vi "StartPythonEventLog.vi"(11 "Console Visibility":T1) -> (3 "Session ID out":T2 format="%x")   [LabVIEW 2018]
uses:
  <vilib>/Enthought/Python Integration Toolkit/api/Session ID.ctl
  <vilib>/Enthought/Python Integration Toolkit/api/Console Visibility.ctl
  Global Variables.vi
  <vilib>/Enthought/Python Integration Toolkit/Python Integration Toolkit.lvlib
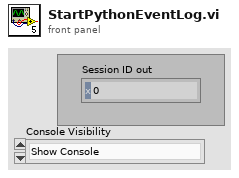
[diagram p1: front panel]
types:
  T1 = typedef "Python Integration Toolkit.lvlib/Console Visibility.ctl" = enum16{"Show Console", "Show Console While Running", "Hide Console"}
  T2 = typedef "Python Integration Toolkit.lvlib/Session ID.ctl" = u64
  T3 = enum16{"open", "replace", "create", "open or create", "replace or create", "replace or create with confirmation"}
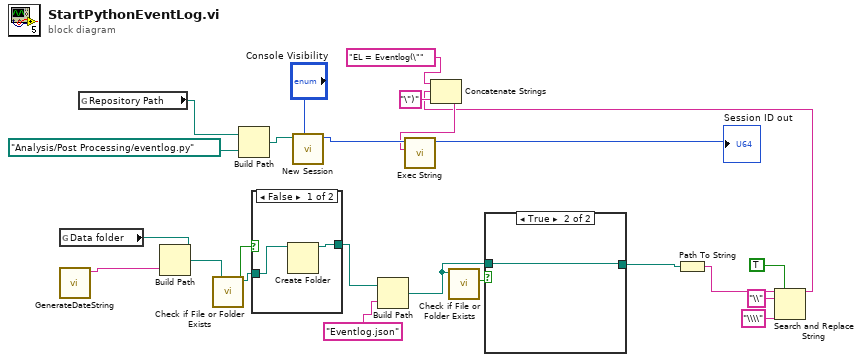
[diagram p0: block diagram]
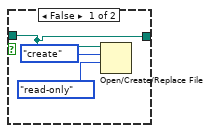
[diagram p2: hidden frame]
diagram:
  n1 = global read "Global Variables.vi" "Data folder"() -> (w18:path)
  n2 = call "GenerateDateString.vi"() -> ("String"=w19:string)  [unwired: 11 in]
  n3 = global read "Global Variables.vi" "Repository Path"() -> (w14:path)
  n4 = Build Path(base path=w18, name or relative path=w19) -> (appended path=w22:path)
  n5 = call <vilib>:"Check if File or Folder Exists.vi"("path"=w22) -> ("file or folder exists?"=w20:bool, "dup path"=w21:path)  [unwired: 8 in, 1 out]
  n6 = Build Path(base path=w14, name or relative path=path "Analysis/Post Processing/eventlog.py" ("vi path")) -> (appended path=w16:path)
  n7 = case shown="False" w20 {
    tunnel: w21 -> [w26 w27]
    tunnel: [w25 w27] -> w23
    frame False {
      n8 = Create Folder(path (use dialog)=w26) -> (created path=w25:path)  [unwired: 2 in, 2 out]
    }
    frame True {
    }
  }
  n9 = call <vilib>:"New Session.vi"("Console Visibility"="Console Visibility", "Path to Python Module (.py File)"=w16) -> ("Session ID out"=w10:T2)  [unwired: 8 in, 1 out]
  n10 = Build Path(base path=w23, name or relative path="Eventlog.json" ("string")) -> (appended path=w12:path)
  n11 = call <vilib>:"Check if File or Folder Exists.vi"("path"=w12) -> ("file or folder exists?"=w13:bool)  [unwired: 8 in, 2 out]
  n12 = case shown="True" w13 {
    tunnel: w12 -> [w30 w31]
    tunnel: [w30 w31] -> w11
    frame False {
      n13 = Open/Create/Replace File(file path (use dialog)=w30, operation (0:open)=T3."create", access (0:read/write)=enum16{"read/write", "read-only", "write-only"}."read-only") -> ()  [unwired: 3 in, 3 out]
    }
    frame True {
    }
  }
  n14 = Path To String(path=w11) -> (string=w5:string)
  n15 = Search and Replace String(replace all?=TRUE ("replace all? (F)"), input string=w5, search string="\\", replace string="\\\\" ("replace string (\"\")")) -> (result string=w2:string)  [unwired: 4 in, 3 out]
  n16 = Concatenate Strings("EL = Eventlog(\"" ("Python Code"), w2, "\")" ("string")) -> (w6:string)
  n17 = call <vilib>:"Exec String.vi"("Python Code"=w6, "Session ID"=w10) -> ("Session ID out"=→"Session ID out":T2)  [unwired: 8 in, 1 out]
